vi "CmdControl.vi"() -> (1 "Dataout":u8[](array[numeric]))   [LabVIEW 2010]
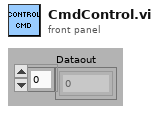
[diagram p1: front panel]
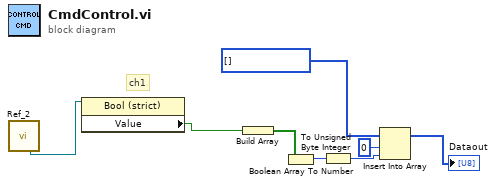
[diagram p0: block diagram]
diagram:
  # "ch1"
  n1 = call "Ref_2.vi"() -> ("Control  Ch 1 out"=w6:refnum<vi>)  [unwired: 17 in, 10 out]
  n2 = property class="Bool (strict)"(reference=w6) -> ("Value"=w5:bool)  [unwired: 1 in, 2 out]
  n3 = Build Array(w5) -> (w4:bool[])
  n4 = Boolean Array To Number(Boolean array=w4) -> (number=w3:u32)
  n5 = To Unsigned Byte Integer(number=w3) -> (unsigned 8bit integer=w2:u8)
  n6 = Insert Into Array(array=u8[] [] ("Data 2"), index=0, new element=w2) -> (→"Dataout":u8[])
